vi "To XML - Adds XML Entities.vi"() -> ()   [LabVIEW 2017, in "Cobertura.Tests.lvlib" / "Line.lvlib"]
uses:
  Line.lvlib
  <vilib>/xml/Close Reference(Node).vi
  Cobertura/Line/Line.lvclass
  <vilib>/xml/NI_XML.lvlib
  <resource>/objmgr/DOMUserDefRef.rc
  <vilib>/PNR/Transparent Assertions/Transparent Assertions/Transparent Assertions.lvlib
panel:
  out "error out":errorcluster
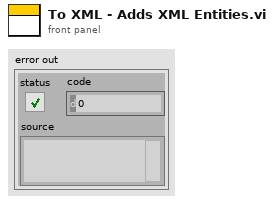
[diagram p1: front panel]
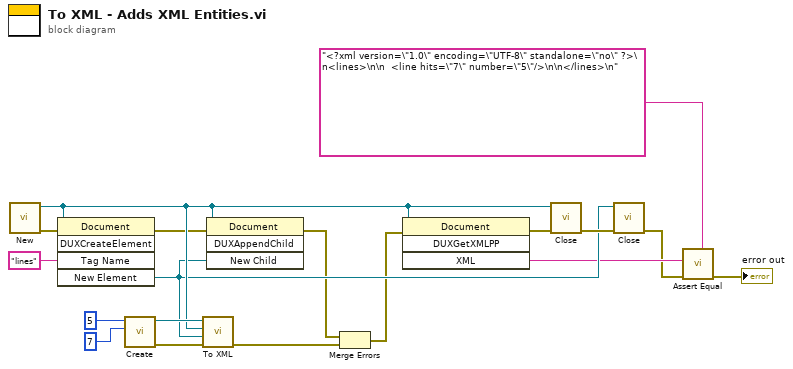
[diagram p0: block diagram]
diagram:
  n1 = call <vilib>:"New.vi"() -> ("error out"=w12:errorcluster, "DOM document out"=w14:refnum<k20>)  [unwired: 8 in]
  n2 = invoke class="Document" method="DUXCreateElement"(reference=w14, error in=w12, "Tag Name"="lines") -> (error out=w13:errorcluster, "New Element"=w10:refnum<k20>)  [unwired: 2 in, 3 out]
  n3 = call "Create.vi"("Hits"=u32 7, "Number"=u32 5) -> ("error out"=w17:errorcluster, "Line"=w18:refnum<class "Line.lvclass">)  [unwired: 8 in]
  n4 = call-dynamic "To XML.vi"("error in (no error)"=w17, "Parent"=w10, "Document"=w14, "Line in"=w18) -> ("error out"=w2:errorcluster)  [unwired: 7 in]
  n5 = invoke class="Document" method="DUXAppendChild"(reference=w14, error in=w13, "New Child"=w10) -> (error out=w4:errorcluster)  [unwired: 1 in, 3 out]
  n6 = Merge Errors(w4, w2) -> (w3:errorcluster)
  n7 = invoke class="Document" method="DUXGetXMLPP"(reference=w14, error in=w3) -> (error out=w15:errorcluster, "XML"=w9:string)  [unwired: 2 in, 2 out]
  n8 = call-poly <vilib>:"Close.vi"("error in (no error)"=w15, "node"=w14) -> ("error out"=w11:errorcluster)  [unwired: 7 in]
  n9 = call-poly <vilib>:"Close.vi"("error in (no error)"=w11, "node"=w10) -> ("error out"=w1:errorcluster)  [unwired: 7 in]
  n10 = call <vilib>:"Assert Equal.vi"("Expected"="<?xml version=\"1.0\" encoding=\"UTF-8\" standalone=\"no\" ?>\n<lines>\n\n  <line hits=\"7\" number=\"5\"/>\n\n</lines>\n", "error in (no error)"=w1, "Actual"=w9) -> ("error out"=→"error out":errorcluster)  [unwired: 8 in]
